vi "Cell V Readback All.vi"(7 "Box ID":u8, 8 "error in (no error)":errorcluster, 11 "ENET in":refnum<class "ENET_BS120x.lvclass">) -> (0 "error out":errorcluster, 2 "Voltage":dbl[](array[numeric]), 3 "ENET out":refnum<class "ENET_BS120x.lvclass">)   [LabVIEW 2021, in "BS120x Driver.lvlib" / "ENET_BS120x.lvclass"]
uses:
  ENET_BS120x.lvclass
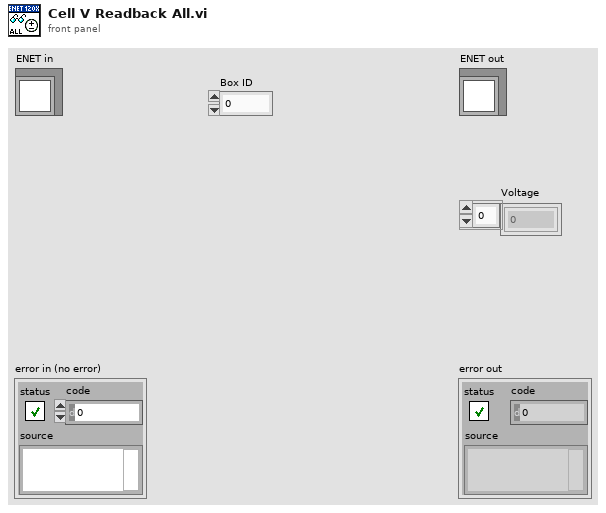
[diagram p1: front panel]
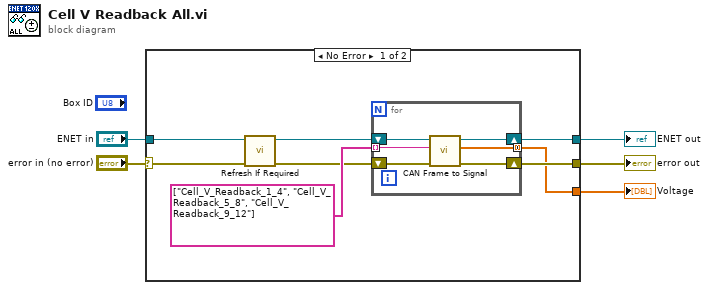
[diagram p0: block diagram]
diagram:
  n1 = case shown="No Error" "error in (no error)" {
    selector: "error in (no error)" -> [w9 w20]
    tunnel: [w12 w20] -> w5
    tunnel: [w11 w21] -> w4
    tunnel: [w10 _] -> w3
    tunnel: "ENET in" -> [w7 w21]
    frame No Error {
      n2 = call "Refresh If Required.vi"("error in (no error)"=w9, "Ethernet in"=w7) -> ("error out"=w8:errorcluster, "Ethernet out"=w6:refnum<class "ENET_BS120x.lvclass">)  [unwired: 8 in]
      n3 = for {
        shift-right: [w16] -> w11
        shift-left: w6 -> [w17]
        tunnel: string[] ["Cell_V_Readback_1_4", "Cell_V_Readback_5_8", "Cell_V_Readback_9_12"] -> [w15] mode=indexing
        tunnel: [w14] -> w10 mode=concatenating
        shift-right: [w18] -> w12
        shift-left: w8 -> [w19]
        n4 = call "CAN Frame to Signal.vi"("error in (no error)"=w19, "Frame"=w15, "ENET in"=w17) -> ("error out"=w18:errorcluster, "signal data"=w14:dbl[], "ENET out"=w16:refnum<class "ENET_BS120x.lvclass">)  [unwired: 6 in]
      }
    }
    frame Error {
    }
  }
  "error out" <- w5
  "ENET out" <- w4
  "Voltage" <- w3
